vi "Set Default RTD Sensor.vi"(8 "error in (no error)":errorcluster, 10 "Default RTD Sensor (0: 100 ohm PT385)":u32(ring) items=["100 ohm PT385", "200 ohm PT385", "500 ohm PT385", "1000 ohm PT385", "PT3926", "PT3916", "CU10", "NI120"], 11 "VISA resource name":refnum<visa-resource-name>) -> (0 "error out":errorcluster, 3 "VISA resource name out":refnum<visa-resource-name>)   [LabVIEW 2011, in "Fluke 5XXX Series Multicalibrators.lvlib"]
doc: "This VI sets the default Resistance Temperature Detector (RTD) at power on and reset, which is saved in the Calibrator non-volatile memory. (While saving configuration data in the non-volatile memory, a period of about 2 seconds, the Calibrator does not respond to remote commands.)\n\nNote:\n\nThis VI is available only for instrument models 5500A and 5520A."
uses:
  Fluke 5XXX Series Multicalibrators.lvlib
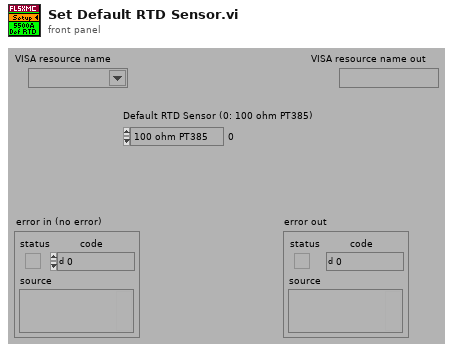
[diagram p1: front panel]
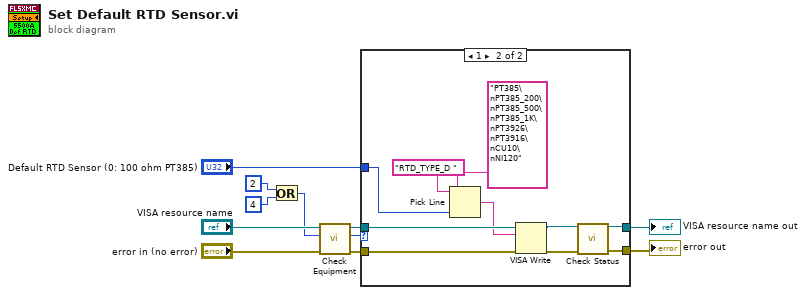
[diagram p0: block diagram]
diagram:
  n1 = Or(x=2 ("Numeric"), y=4 ("Numeric")) -> (x .or. y?=w1:i32)
  n2 = call "Check Equipment.vi"("error in (no error)"="error in (no error)", "Bit Mask"=w1, "VISA resource name"="VISA resource name") -> ("error out"=w11:errorcluster, "Present?"=w10:u32, "VISA resource name out"=w9:refnum<visa-resource-name>)  [unwired: 6 in]
  n3 = case shown="1" w10 {
    tunnel: "Default RTD Sensor (0: 100 ohm PT385)" -> [_ w18]
    tunnel: [w12 w14] -> w5
    tunnel: w11 -> [w13 w21]
    tunnel: w9 -> [w12 w20]
    tunnel: [w13 w17] -> w6
    frame 0, Default {
    }
    frame 1 {
      n4 = Pick Line(string ("")="RTD_TYPE_D " ("Reset Command"), multi-line string="PT385\nPT385_200\nPT385_500\nPT385_1K\nPT3926\nPT3916\nCU10\nNI120", line index=w18) -> (output string=w19:string)
      n5 = VISA Write(VISA resource name=w20, write buffer=w19, error in (no error)=w21) -> (VISA resource name out=w15:refnum<visa-resource-name>, error out=w16:errorcluster)  [unwired: 1 out]
      n6 = call "Check Status.vi"("VISA resource name"=w15, "error in (no error)"=w16) -> ("VISA resource name out"=w14:refnum<visa-resource-name>, "error out"=w17:errorcluster)  [unwired: 12 in]
    }
  }
  "VISA resource name out" <- w5
  "error out" <- w6
